vi "StartIclExeViaCommandLine.vi"(8 "error in (no error)":errorcluster, 11 "run minimized?":bool) -> (0 "error out":errorcluster)   [LabVIEW 2020, in "horiba.lvlib" / "DeviceManager.lvlib"]
uses:
  DeviceManager.lvlib
panel:
  # "Connector Pane"
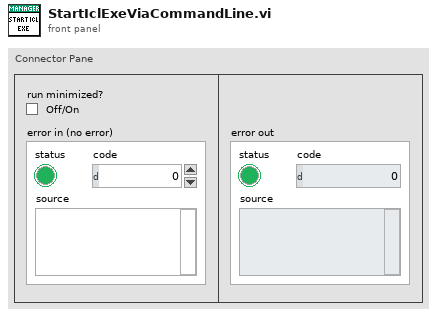
[diagram p1: front panel]
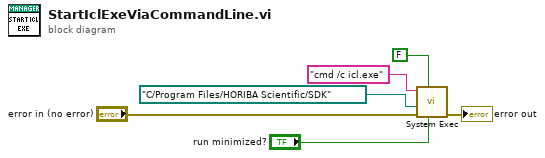
[diagram p0: block diagram]
diagram:
  n1 = call <vilib>:"System Exec.vi"("run minimized? (F)"="run minimized?", "wait until completion? (T)"=FALSE, "error in (no error)"="error in (no error)", "working directory"=path "C:/Program Files/HORIBA Scientific/SDK", "command line"="cmd /c icl.exe") -> ("error out"=→"error out":errorcluster)  [unwired: 3 in, 3 out]
